vi "SelectFileType.vi"() -> (1 "ExportedFilePath":path, 2 "FileType":enum16{"None", "CSV", "XLS"}(ring))   [LabVIEW 2024]
panel:
  in  "SaveAsXls":bool
  in  "SaveAsCSV":bool
  in  "Cancel Button":bool
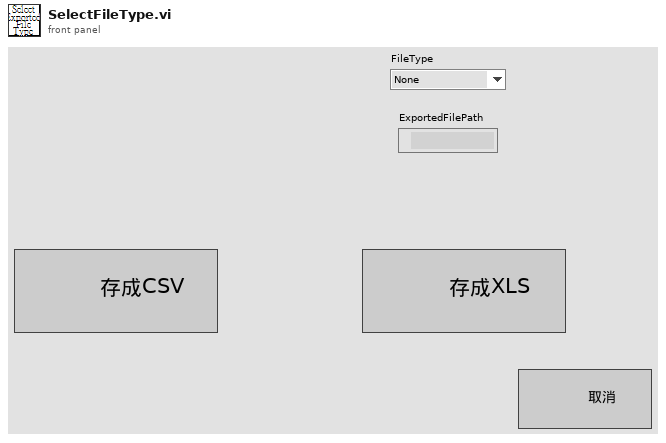
[diagram p1: front panel]
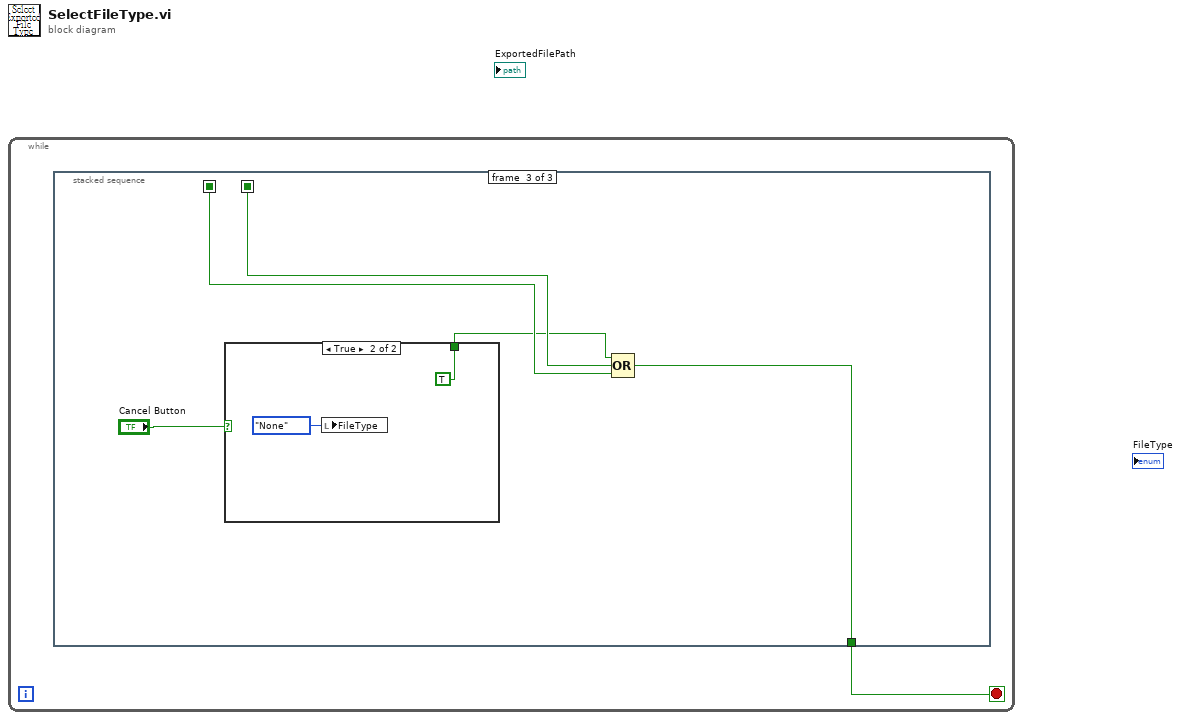
[diagram p0: block diagram]
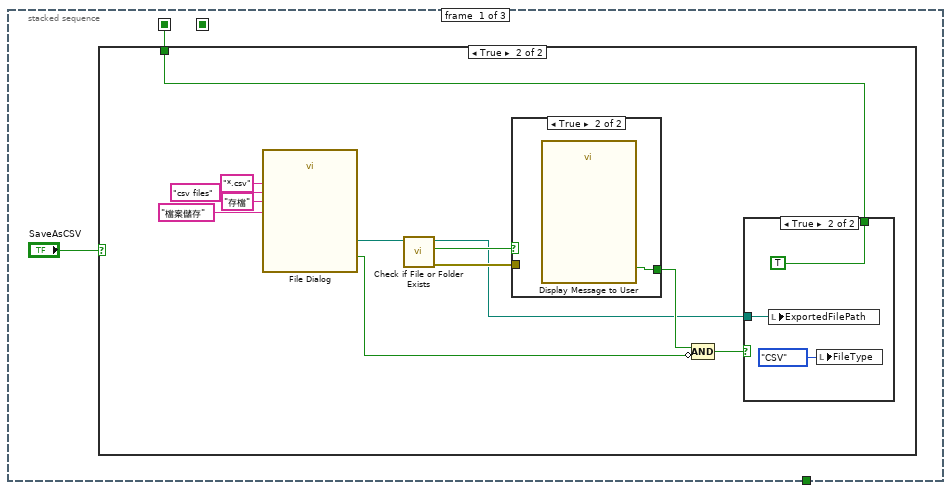
[diagram p2: hidden frame]
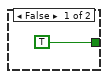
[diagram p5: hidden frame]
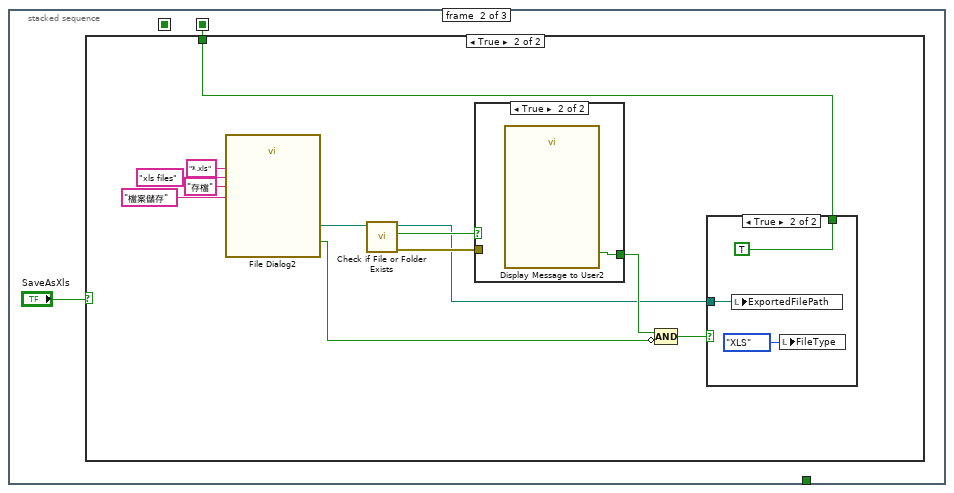
[diagram p6: hidden frame]
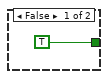
[diagram p9: hidden frame]
diagram:
  n1 = while {
    stop <- w1 stop-if-true
    n2 = stacked-sequence {
      seq-local: [w2 _ _] -> [_ _ w43]
      seq-local: [_ w21 _] -> [_ _ w42]
      tunnel: [_ _ w40] -> w1
      frame #0 {
        n3 = case shown="True" "SaveAsCSV" {
          tunnel: [_ w4] -> w2
          frame False {
          }
          frame True {
            n4 = call "File Dialog"("prompt"="檔案儲存", "button label"="存檔", "pattern (all files)"="*.csv", "pattern label"="csv files") -> ("selected path"=w9:path, "cancelled"=w8:bool)  [unwired: 8 in, 2 out]
            n5 = call <vilib>:"Check if File or Folder Exists.vi"("path"=w9) -> ("error out"=w10:errorcluster, "file or folder exists?"=w11:bool, "dup path"=w5:path)  [unwired: 8 in]
            n6 = case shown="True" w11 {
              tunnel: [TRUE w20] -> w7
              tunnel: w10 -> [_ _]
              frame False {
              }
              frame True {
                n7 = call "Display Message to User"() -> ("YES"=w20:bool)  [unwired: 10 in, 1 out]
              }
            }
            n8 = Compound Arithmetic op=AND(w7, invert w8) -> (w6:bool)
            n9 = case shown="True" w6 {
              tunnel: w5 -> [_ w18]
              tunnel: [_ TRUE] -> w4
              frame False {
              }
              frame True {
                n10 = local write "ExportedFilePath"(w18) -> ()
                n11 = local write "FileType"(enum16{"None", "CSV", "XLS"}."CSV" ("FileType")) -> ()
              }
            }
          }
        }
      }
      frame #1 {
        n12 = case shown="True" "SaveAsXls" {
          tunnel: [_ w23] -> w21
          frame False {
          }
          frame True {
            n13 = call "File Dialog2"("prompt"="檔案儲存", "button label"="存檔", "pattern (all files)"="*.xls", "pattern label"="xls files") -> ("selected path"=w28:path, "cancelled"=w27:bool)  [unwired: 8 in, 2 out]
            n14 = call <vilib>:"Check if File or Folder Exists.vi"("path"=w28) -> ("error out"=w29:errorcluster, "file or folder exists?"=w30:bool, "dup path"=w24:path)  [unwired: 8 in]
            n15 = case shown="True" w30 {
              tunnel: [TRUE w39] -> w26
              tunnel: w29 -> [_ _]
              frame False {
              }
              frame True {
                n16 = call "Display Message to User2"() -> ("YES"=w39:bool)  [unwired: 10 in, 1 out]
              }
            }
            n17 = Compound Arithmetic op=AND(w26, invert w27) -> (w25:bool)
            n18 = case shown="True" w25 {
              tunnel: w24 -> [_ w37]
              tunnel: [_ TRUE] -> w23
              frame False {
              }
              frame True {
                n19 = local write "ExportedFilePath"(w37) -> ()
                n20 = local write "FileType"(enum16{"None", "CSV", "XLS"}."XLS" ("FileType")) -> ()
              }
            }
          }
        }
      }
      frame #2 {
        n21 = case shown="True" "Cancel Button" {
          tunnel: [_ TRUE] -> w41
          frame False {
          }
          frame True {
            n22 = local write "FileType"(enum16{"None", "CSV", "XLS"}."None" ("FileType")) -> ()
          }
        }
        n23 = Compound Arithmetic op=OR(w41, w42, w43) -> (w40:bool)
      }
    }
  }
